vi "Set User Event.vi"(8 "error in (no error)":errorcluster, 11 "userEvent":u32) -> (0 "error out":errorcluster, 2 "function return":u32, 3 "userEvent out":u32)   [LabVIEW 2014, in "atmcd32d.lvlib"]
doc: "unsigned int WINAPI SetUserEvent(HANDLE userEvent);"
uses:
  atmcd32d.lvlib
  atmcd32d.dll
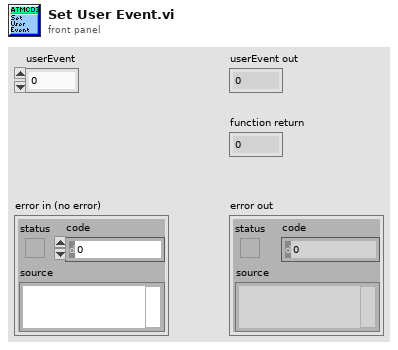
[diagram p1: front panel]
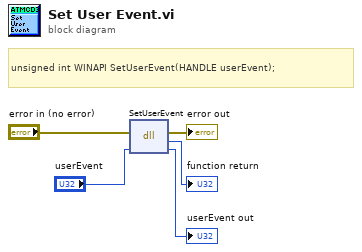
[diagram p0: block diagram]
diagram:
  # "unsigned int WINAPI SetUserEvent(HANDLE userEvent);"
  n1 = dll-call lib="C:/Users/Bakir/Documents/Lambda2-Testing/lib/Andorlib/atmcd32d.*" fn="SetUserEvent"(error in="error in (no error)", "userEvent"="userEvent") -> (error out=→"error out":errorcluster, →"function return":u32, "userEvent"=→"userEvent out":u32)  [unwired: 2 in, 1 out]
